vi "BRig_RT__Case_Exp__storeData__endExp__v5__p3.vi"(7 "input_True":bool=TRUE, 9 "input_dataAnalog":u16[][](array[numeric]), 11 "input_dataAnalog_length":i32) -> (8 "output_True":bool)   [LabVIEW 2014]
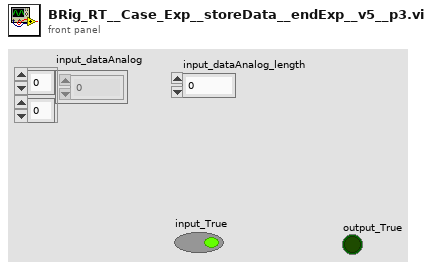
[diagram p1: front panel]
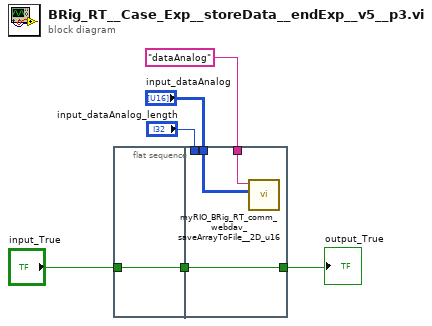
[diagram p0: block diagram]
diagram:
  n1 = flat-sequence {
    tunnel: [w7] -> w3
    tunnel: "input_True" -> [w7]
    tunnel: "input_dataAnalog_length" -> [_]
    tunnel: "input_dataAnalog" -> [w8]
    tunnel: "dataAnalog" ("input_filename") -> [w10]
    tunnel: w3 -> [w9]
    tunnel: [w9] -> w2
    frame #0 {
    }
    frame #1 {
      n2 = call "myRIO_BRig_RT_comm_webdav_saveArrayToFile__2D_u16.vi"("Array"=w8, "input_filename"=w10) -> ()  [unwired: 10 in]
    }
  }
  "output_True" <- w2
